vi "Get Inventory Data.vi"(8 "error in (no error)":errorcluster) -> (0 "error out":errorcluster, 3 "Array":T1[](array[typedef]))   [LabVIEW 2020, in "SQLITE Inventory.lvlib"]
uses:
  SQLITE Inventory.lvlib
  Invetory Data Type.ctl
  <vilib>/drjdpowell/SQLite Library/SQL Connection/Open (path).vi
  <vilib>/drjdpowell/SQLite Library/SQL Connection/Open (string).vi
  <vilib>/AdvancedString/Path To Command Line String.vi
  <vilib>/drjdpowell/SQLite Library/SQL Connection/Execute SQL (1D String).vi
  <vilib>/drjdpowell/SQLite Library/SQL Connection/Execute SQL (Single Integer).vi
  <vilib>/drjdpowell/SQLite Library/SQL Connection/Connection.lvclass
  <vilib>/drjdpowell/SQLite Library/SQLite.lvlib
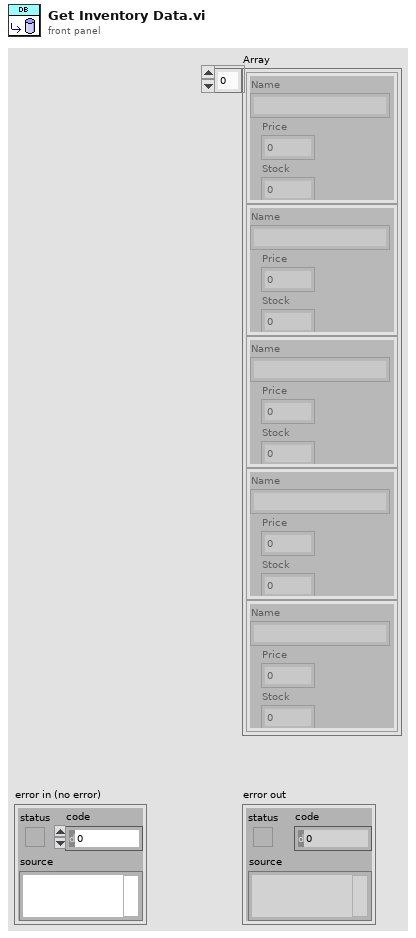
[diagram p1: front panel]
types:
  T1 = typedef "Invetory Data Type.ctl" = cluster{"Name":string, "Price":dbl, "Stock":dbl}
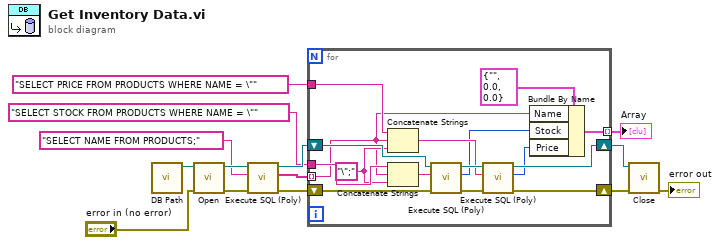
[diagram p0: block diagram]
diagram:
  n1 = call "DB Path.vi"() -> ("DB Path"=w12:path)  [unwired: 11 in]
  n2 = call-poly <vilib>:"Open.vi"("error in (no error)"="error in (no error)", "db file"=w12) -> ("error out"=w14:errorcluster, "SQLite Connection"=w13:refnum<class "Connection.lvclass">)  [unwired: 8 in]
  n3 = call-poly <vilib>:"Execute SQL (Poly).vi"("error in (no error)"=w14, "SQL"="SELECT NAME FROM PRODUCTS;", "SQLite Connection in"=w13) -> ("error out"=w9:errorcluster, "Result Set"=w6:string[], "SQLite Connection"=w10:refnum<class "Connection.lvclass">)  [unwired: 5 in, 1 out]
  n4 = for {
    shift-right: [w27] -> w8
    shift-left: w10 -> [w30]
    shift-right: [w28] -> w7
    shift-left: w9 -> [w29]
    tunnel: w6 -> [w17] mode=indexing
    tunnel: "SELECT STOCK FROM PRODUCTS WHERE NAME = \"" ("SQL") -> [w26]
    tunnel: "SELECT PRICE FROM PRODUCTS WHERE NAME = \"" ("SQL") -> [w21]
    tunnel: [w18] -> w3 mode=indexing
    w22 = "\";"
    n5 = Concatenate Strings(w21, w17, w22) -> (w20:string)
    n6 = Concatenate Strings(w26, w17, w22) -> (w23:string)
    n7 = call-poly <vilib>:"Execute SQL (Poly).vi"("error in (no error)"=w29, "SQL"=w23, "SQLite Connection in"=w30) -> ("error out"=w25:errorcluster, "Result"=w16:i64, "SQLite Connection"=w24:refnum<class "Connection.lvclass">)  [unwired: 6 in]
    n8 = call-poly <vilib>:"Execute SQL (Poly).vi"("error in (no error)"=w25, "SQL"=w20, "SQLite Connection in"=w24) -> ("error out"=w28:errorcluster, "Result"=w15:i64, "SQLite Connection"=w27:refnum<class "Connection.lvclass">)  [unwired: 6 in]
    n9 = Bundle By Name(cluster=T1 {"Name"="", "Price"=0.0, "Stock"=0.0}, "Name"=w17, "Stock"=w16, "Price"=w15) -> (w18:T1)
  }
  "Array" <- w3
  n10 = call-dynamic "Close.vi"("error in (no error)"=w7, "SQLite Connection in"=w8) -> ("error out"=→"error out":errorcluster)  [unwired: 9 in]
